vi "SENS_IF_FILT_STAGE_COEF.vi"(0 "VISA IN":refnum<visa-resource-name>, 1 "Stage number":i32, 2 "Filter Coefficients":string, 5 "error in":errorcluster, 7 "Channel":i32) -> (14 "VISA Out":refnum<visa-resource-name>, 19 "error out":errorcluster)   [LabVIEW 2018, in "PNA-X.lvlib"]
doc: "SENSe<cnum>:IF:FILTer:STAGE<n>:COEFficients <coef> \n1755\n\n(Read-Write) Sets and returns the digital filter coefficients of the specified stage. \nCritical Note \nParameters \n<cnum> Existing channel number. If unspecified, <cnum> is set to 1. \n<n> Stage number. Choose 1 or 2 \n<coef> An array of real numbers. Filter coefficients \nExamples SENS:IF:FILT:STAG2:COEF 0,0.1,0.7,0.7,0.1 \nsense2:if:filter:stage1:coefficients \nQuery Syntax SENSe<cnum>:IF:FILTer:STAGE<n>:COEFficients? \nExample SENS:IF:FILT:STAG2:COEF? \nsense2:if:filter:stage1:coefficients? \nReturn Type Numeric \nDefault Stage dependent"
uses:
  PNA-X.lvlib
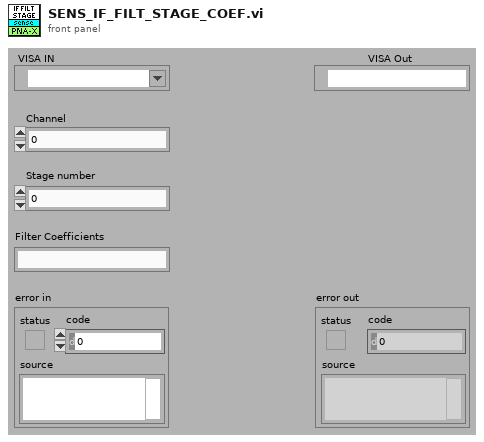
[diagram p1: front panel]
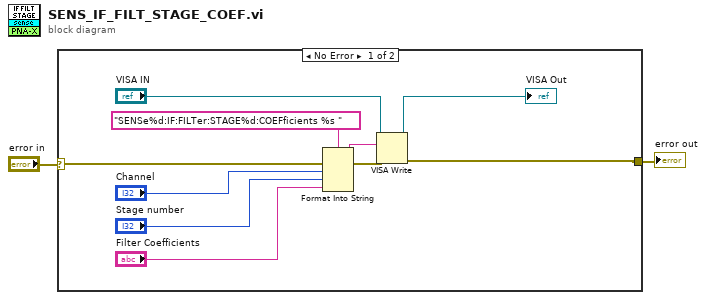
[diagram p0: block diagram]
diagram:
  n1 = case shown="No Error" "error in" {
    selector: "error in" -> [w12 w13]
    tunnel: [w7 w13] -> w1
    frame No Error {
      n2 = Format Into String(format string="SENSe%d:IF:FILTer:STAGE%d:COEFficients %s " ("Cmdline"), error in=w12, "Channel", "Stage number", "Filter Coefficients") -> (resulting string=w10:string, error out=w11:errorcluster)  [unwired: 1 in]
      n3 = VISA Write(VISA resource name="VISA IN", write buffer=w10, error in (no error)=w11) -> (VISA resource name out=→"VISA Out":refnum<visa-resource-name>, error out=w7:errorcluster)  [unwired: 1 out]
    }
    frame Error {
    }
  }
  "error out" <- w1
